vi "33_stretch_strengthening.vi"() -> ()   [LabVIEW 2018]
uses:
  <vilib>/vision/NI_Vision_Development_Module.lvlib
panel:
  in  "adj":dbl(slide)=255.0 scale=0.0..1000.0
  out "new":T1(plugin-control)
  out "Array":u8[][](array[numeric])
  out "Image 2":T1(plugin-control)
  out "Image Pixels (U8)":u8[][](array[numeric])
  in  "stop":bool
  out "Image":T1(plugin-control)
  # "拉伸強化"
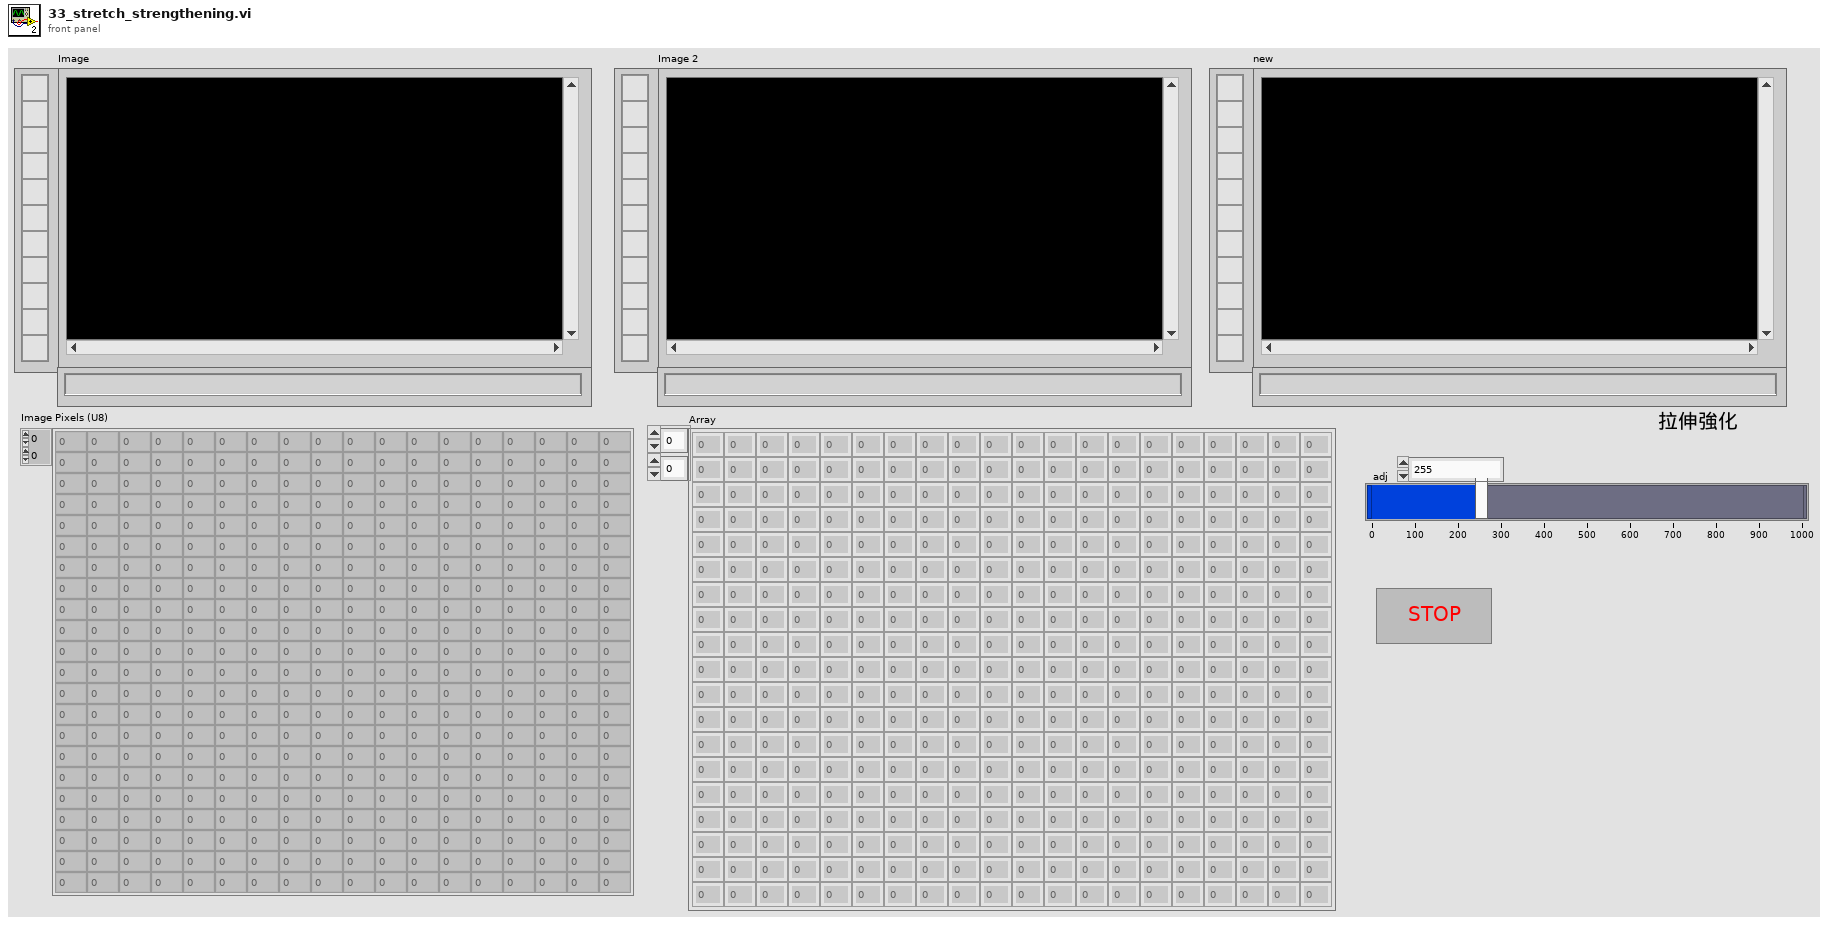
[diagram p1: front panel]
types:
  T1 = typedef "IMAQ Image.ctl" = refnum<image>
  T2 = typedef "Image Type" = u32
  T3 = cluster{"Global Rectangle":i32[], "Contours":cluster{"Contour Type":u32, "ROI Type":u32, "Points":i32[]}[]}
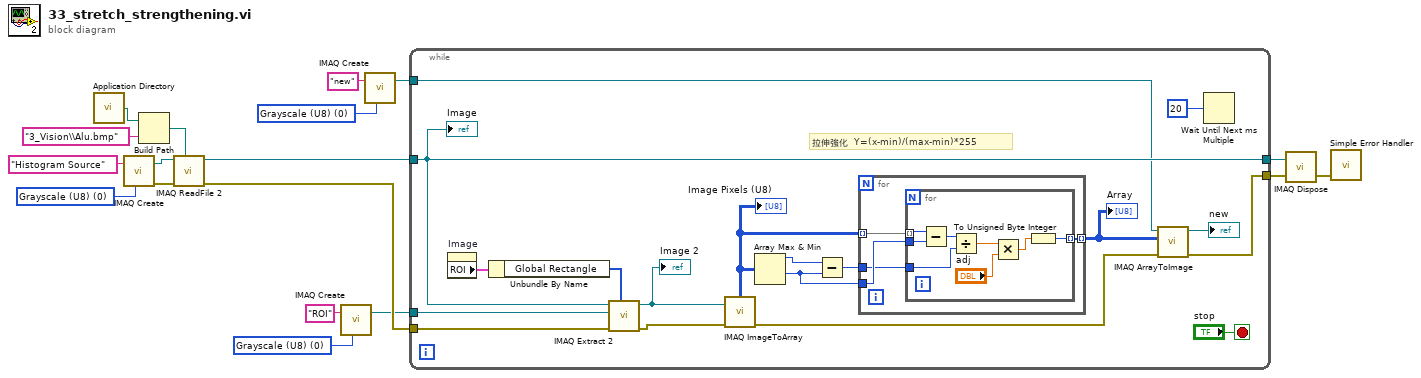
[diagram p0: block diagram]
diagram:
  w2 = T2 0 items=["Grayscale (U8)", "Grayscale (I16)", "Grayscale (SGL)", "Complex (CSG)", "RGB (U32)", "HSL (U32)", "RGB (U64)", "Grayscale (U16)"] ("Image Type")
  w7 = T2 0 items=["Grayscale (U8)", "Grayscale (I16)", "Grayscale (SGL)", "Complex (CSG)", "RGB (U32)", "HSL (U32)", "RGB (U64)", "Grayscale (U16)"] ("Image Type")
  w8 = T2 0 items=["Grayscale (U8)", "Grayscale (I16)", "Grayscale (SGL)", "Complex (CSG)", "RGB (U32)", "HSL (U32)", "RGB (U64)", "Grayscale (U16)"] ("Image Type")
  n1 = call <vilib>:"Application Directory.vi"() -> ("Application Directory"=w10:path)
  n2 = call "IMAQ Create"("Image Name"="Histogram Source", "Image Type"=w8) -> ("New Image"=w18:T1, "error out"=w17:errorcluster)  [unwired: 3 in]
  n3 = Build Path(base path=w10, name or relative path="3_Vision\\Alu.bmp") -> (appended path=w11:path)
  n4 = call "IMAQ ReadFile 2"("File Path"=w11, "error in (no error)"=w17, "Image"=w18) -> ("error out"=w13:errorcluster, "Image Out"=w15:T1)  [unwired: 4 in, 3 out]
  n5 = call "IMAQ Create"("Image Name"="ROI", "Image Type"=w7) -> ("New Image"=w5:T1)  [unwired: 3 in, 1 out]
  n6 = call "IMAQ Create"("Image Name"="new", "Image Type"=w2) -> ("New Image"=w1:T1)  [unwired: 3 in, 1 out]
  n7 = while {
    tunnel: w15 -> [w33]
    tunnel: [w33] -> w14
    tunnel: w13 -> [w30]
    tunnel: w5 -> [w32]
    tunnel: [w23] -> w4
    tunnel: w1 -> [w26]
    stop <- "stop" stop-if-true
    # "拉伸強化  Y=(x-min)/(max-min)*255"
    n8 = property on="Image" class="ImageControl"() -> ("ROI"=w34:T3)  [unwired: 2 in, 2 out]
    n9 = Unbundle By Name "Unbundle By Name"(w34) -> ("Global Rectangle"=w31:i32[])
    n10 = call "IMAQ Extract 2"("Optional Rectangle"=w31, "error in (no error)"=w30, "Image Dst"=w32, "Image Src"=w33) -> ("error out"=w28:errorcluster, "Image Dst Out"=w29:T1)  [unwired: 6 in]
    "Image 2" <- w29
    n11 = call "IMAQ ImageToArray"("error in (no error)"=w28, "Image"=w29) -> ("error out"=w24:errorcluster, "Image Pixels (U8)"=w22:u8[][])  [unwired: 2 in, 3 out]
    "Image Pixels (U8)" <- w22
    n12 = Array Max & Min(array=w22) -> (max value=w21:u8, min value=w20:u8)  [unwired: 2 out]
    n13 = Subtract(x=w21, y=w20) -> (x-y=w19:u8)
    n14 = for {
      tunnel: w22 -> [w40] mode=indexing
      tunnel: [w39] -> w27 mode=indexing
      tunnel: w20 -> [w38]
      tunnel: w19 -> [w37]
      n15 = for {
        tunnel: w40 -> [w46] mode=indexing
        tunnel: [w41] -> w39 mode=indexing
        tunnel: w38 -> [w45]
        tunnel: w37 -> [w44]
        n16 = Subtract(x=w46, y=w45) -> (x-y=w48:u8)
        n17 = Divide(x=w48, y=w44) -> (x/y=w47:dbl)
        n18 = Multiply(x=w47, y="adj") -> (x*y=w42:dbl)
        n19 = To Unsigned Byte Integer(number=w42) -> (unsigned 8bit integer=w41:u8)
      }
    }
    "Array" <- w27
    n20 = call "IMAQ ArrayToImage"("error in (no error)"=w24, "Image Pixels (U8)"=w27, "Image"=w26) -> ("error out"=w23:errorcluster, "Image Out"=→"new":T1)  [unwired: 7 in]
    n21 = Wait Until Next ms Multiple(millisecond multiple=u32 20) -> ()  [unwired: 1 out]
    "Image" <- w33
  }
  n22 = call "IMAQ Dispose"("Image"=w14, "error in (no error)"=w4) -> ("error out"=w12:errorcluster)  [unwired: 4 in]
  n23 = call <vilib>:"Simple Error Handler.vi"("error in (no error)"=w12) -> ()  [unwired: 4 in, 5 out]
